vi "Version to String.vi"(11 "Version":T1) -> (3 "Version String":string)   [LabVIEW 2020]
uses:
  Version.ctl
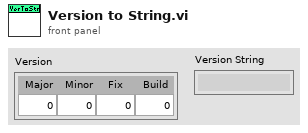
[diagram p1: front panel]
types:
  T1 = typedef "Version.ctl" = cluster{"Major":u16, "Minor":u16, "Fix":u16, "Build":u16}
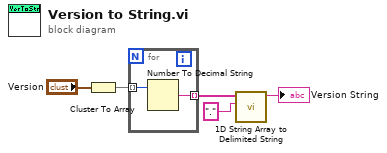
[diagram p0: block diagram]
diagram:
  n1 = Cluster To Array(cluster="Version") -> (array=w4:u16[])
  n2 = for {
    tunnel: w4 -> [w7] mode=indexing
    tunnel: [w6] -> w3 mode=indexing
    n3 = Number To Decimal String(number=w7) -> (decimal integer string=w6:string)  [unwired: 1 in]
  }
  n4 = call <vilib>:"1D String Array to Delimited String.vi"("delimiter"=".", "string array"=w3) -> ("delimited string"=→"Version String":string)  [unwired: 9 in]
